vi "SIT_Limit Display.vi"(9 "Limit":i32=100, 11 "Data In":string) -> (1 "Line Count":i32, 3 "Data Out":string)   [LabVIEW 2010]
panel:
  in  "String":string
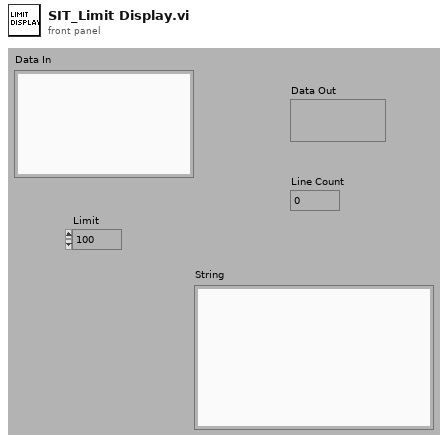
[diagram p1: front panel]
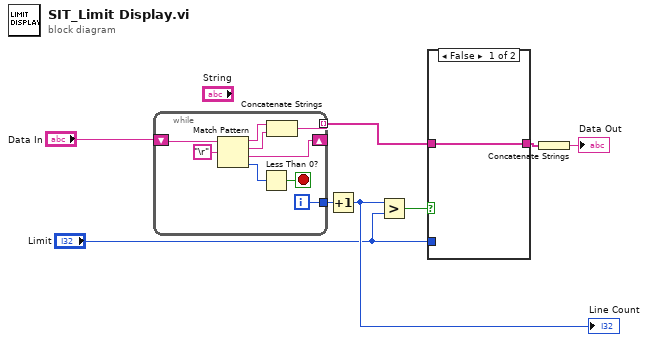
[diagram p0: block diagram]
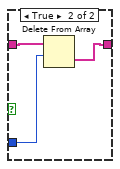
[diagram p2: hidden frame]
diagram:
  n1 = while {
    tunnel: [w15] -> w8
    tunnel: [w11] -> w4 mode=indexing
    shift-right: [w9] -> _
    shift-left: "Data In" -> [w17]
    i -> [w15]
    stop <- w16 stop-if-true
    n2 = Match Pattern(string=w17, regular expression="\r") -> (before substring=w10:string, match substring=w12:string, after substring=w9:string, offset past match=w14:i32)  [unwired: 1 in]
    n3 = Less Than 0?(x=w14) -> (x < 0?=w16:bool)
    n4 = Concatenate Strings(w10, w12) -> (w11:string)
  }
  n5 = Increment(x=w8) -> (x+1=w6:i32)
  "Line Count" <- w6
  n6 = Greater?(x=w6, y="Limit") -> (0:w5:bool)
  n7 = case shown="False" w5 {
    tunnel: w4 -> [w18 w21]
    tunnel: [w18 w19] -> w2
    tunnel: "Limit" -> [_ w20]
    frame False {
    }
    frame True {
      n8 = Delete From Array(array=w21, length=w20) -> (deleted portion=w19:string[])  [unwired: 1 in, 1 out]
    }
  }
  n9 = Concatenate Strings(w2) -> (→"Data Out":string)
